vi "crio_RT_Antagonist_Precision.vi"() -> ()   [LabVIEW 2019]
uses:
  <vilib>/Platform/TimedLoop/XDataNode/timing_clust.ctl
  <vilib>/Platform/TimedLoop/XDataNode/nitl_modes.ctl
  <vilib>/Platform/TimedLoop/XDataNode/wakeup.ctl
  <vilib>/FPGAPlugInAG/cRIO-9074/niLvFpga_Open_cRIO-9074.vi
  <vilib>/rvi/interface/common/dynamic/niFpgaDynamicAddResources.vi
  <vilib>/Utility/file.llb/Write Delimited Spreadsheet (string).vi
  <vilib>/Utility/error.llb/Error Cluster From Error Code.vi
  <vilib>/rvi/errors/niLvFpgaAdjustHostInterfaceError.vi
  <vilib>/FPGAPlugInAG/Dynamic/niLvFpga_Close_Dynamic.vi
  <vilib>/rvi/interface/nirviOpenFPGA/nirviOpenFPGA.xnode
  FPGA Bitfiles/gpass2_FPGATarget2_crioFPGAAntagoni_cDOKBUczdNQ.lvbitx
  crio_FPGA_Antagonist_Radial.vi
  <vilib>/rvi/interface/nirviReadWriteControl/nirviReadWriteControl.xnode
  <vilib>/platform/TimedLoop/XDataNode/XDataNode.xnode
  <vilib>/rvi/interface/nirviCloseFPGA/nirviCloseFPGA.xnode
  NiFpgaLv.dll
  <vilib>/rvi/interface/Simulation/niFpgaSimulationCallBeginRW.vi
  <vilib>/Platform/TimedLoop/XDataNode/XDNodeRunTimeDep.lvlib
  <vilib>/Utility/file.llb/Write Delimited Spreadsheet (I64).vi
panel:
  out "appended array":i32[](array[numeric])
  in  "precision test .csv name":string="precision_test.csv"
  in  "Channel Names":string[](array[string])=["Channel 1", "Channel 2", "Channel 3", "Channel 4", "Channel 5"]
  out "log file path":path
  out "error out":errorcluster
  in  "Header Info":string[][](array[string])=[["Test Name", "Operator", "UUT"], ["Voltage", "National Instruments", "AA123"]]
  in  "mSec to take Sample":u32
  in  "LAC Full Extract Position":i32(slide) scale=0.0..4500.0
  in  "VCA Full Extract Position":i32(slide) scale=0.0..2700.0
  in  "Rail Full Extract Position":i16(slide) scale=0.0..20000.0
  out "VCA Setpoint":i32
  out "Rail Setpoint":i16
  out "LAC Setpoint":i32
  in  "Start Test":bool
  out "Rail Position":i16(graph)
  out "rail Platform Position":i16
  in  "Half Peirod (pulse 40MHz)":u32=10000
  in  "Rail Stepper Direction":bool
  in  "Rail Stepper Enable":bool
  in  "Rail Manual Operation":bool
  in  "Autolock":bool
  out "LAC Measured Position":i32(graph)
  out "LAC Measured Position":i32
  in  "LAC manual control":T1={"manual? (F)"=FALSE, "manual input (0)"=-0.83838385} {"manual input (0)" scale=-1.0..1.0}
  in  "LAC Position Reset":bool
  in  "LAC Gains":T2={"proportional gain"=0.95454544, "integral gain"=0.4949495} {"proportional gain" scale=0.0..1.0; "integral gain" scale=0.0..1.0}
  in  "LAC Velocity Interval (uSec)":u32=1000
  out "LAC Actual Gain":T2={"proportional gain"=0.009545455, "integral gain"=1.2626262e-09}
  in  "LAC Gain Scaler":T2={"proportional gain"=100.0, "integral gain"=100000000.0}
  in  "stop":bool
  out "VCA Measured Velocity (Counts/Interval)":i32
  out "VCA Controller PWM Output":sgl=-0.35149753
  out "VCA Measured Position":i32=4
  in  "VCA Loop Period(us)":i64=2000
  out "VCA Measured Position":i32(graph)=4
  in  "VCA  manual control":T1 {"manual input (0)" scale=-1.0..1.0}
  in  "VCA Position Reset":bool
  in  "VCA Gains":T2={"proportional gain"=0.97979796, "integral gain"=0.7979798} {"proportional gain" scale=0.0..1.0; "integral gain" scale=0.0..1.0}
  in  "VCA Velocity Interval (uSec)":u32=1000
  out "VCA Actual Gain":T2={"proportional gain"=0.0009797979, "integral gain"=7.979798e-09}
  in  "VCA Gain Scaler":T2={"proportional gain"=1000.0, "integral gain"=100000000.0}
  in  "PWM Frequency (default 20kHz)":i32=20000
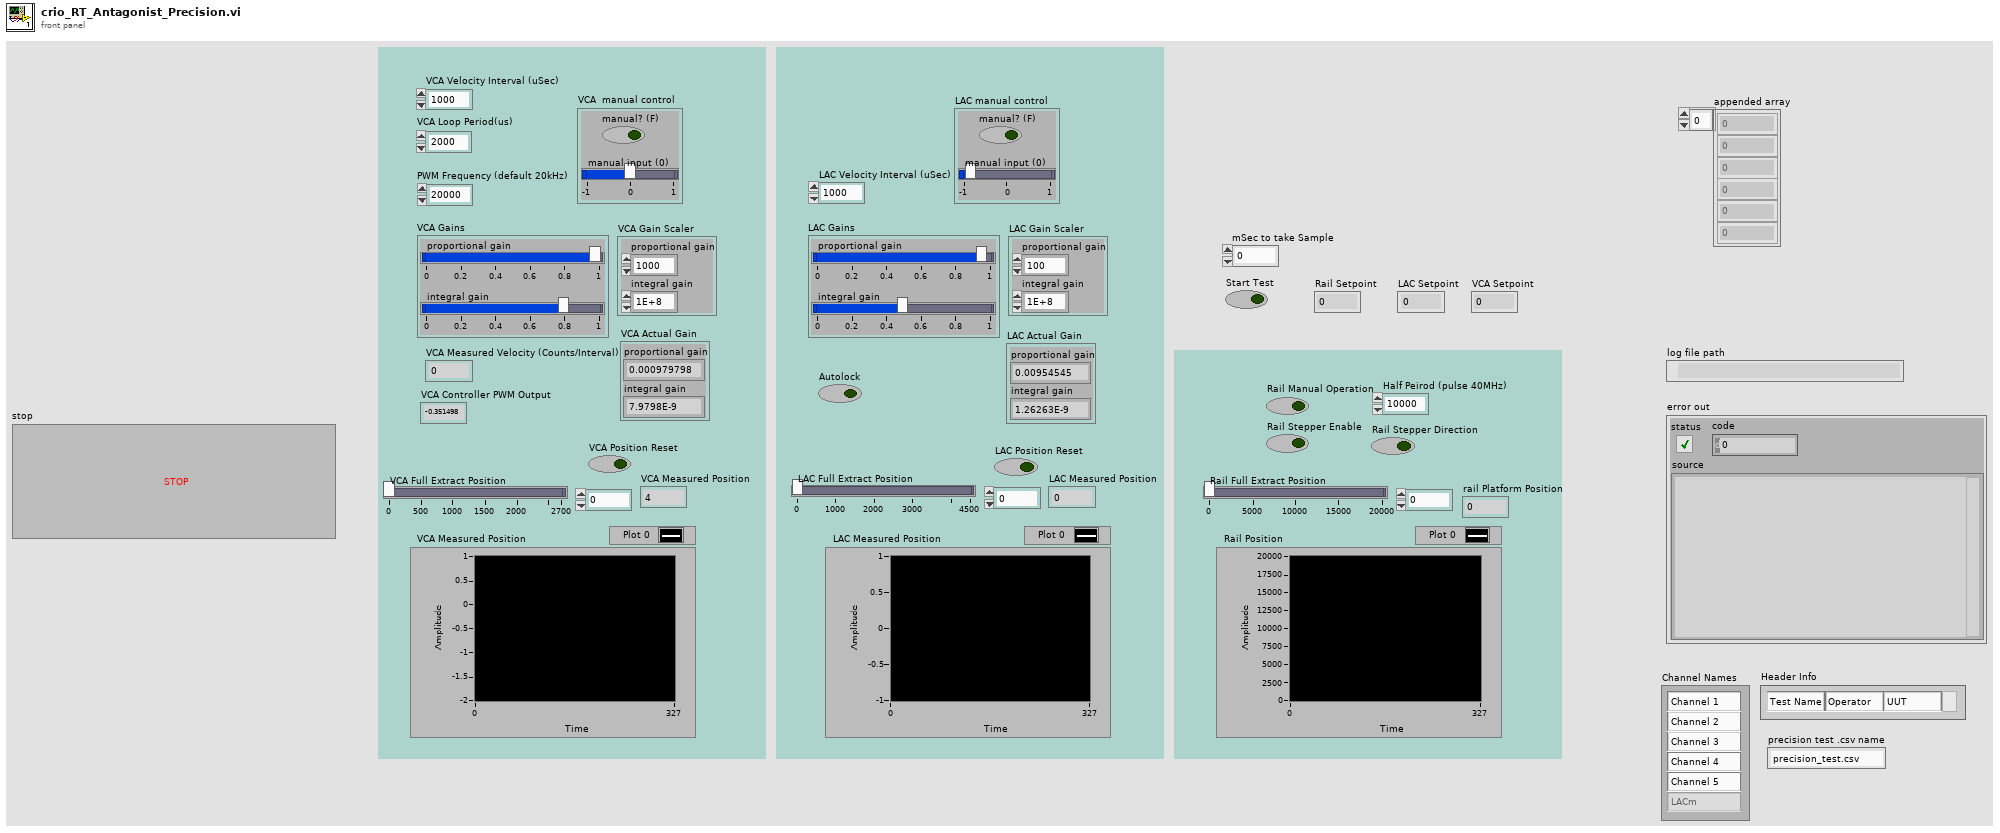
[diagram p1: front panel]
types:
  T1 = cluster{"manual? (F)":bool, "manual input (0)":sgl}
  T2 = cluster{"proportional gain":sgl, "integral gain":sgl}
  T3 = typedef "XDNodeRunTimeDep.lvlib/timing_clust.ctl" = cluster{"Expected End [f-1]":u64, "Actual End [f-1]":u64, "Finished Late? [f-1]":bool, "Expected End [i-1]":u64, "Actual End [i-1]":u64, "Finished Late? [i-1]":bool, "Expected Start [i]":u64, "Actual Start [i]":u64, "Expected Start [f]":u64, "Actual Start [f]":u64, "Source Name":string, "Structure Name":string, "Period":i64, "Deadline":i64, "Offset":i64, "Start":i64, "Priority":i32, "Timeout":i32, "Mode":T4, "Wakeup Reason":T5, "Error":errorcluster, "Source Type":string, "Secondary Source Type":string, "Global End Time":u64, "Global Start Time":u64, "Frame Duration":u64, "Iteration Duration":u64, "Assigned CPU":i32, "I/O Scan Engine Mode":u32}
  T4 = typedef "XDNodeRunTimeDep.lvlib/nitl_modes.ctl" = enum32{"No Change", "Process missed periods, maintain original phase", "Discard missed periods, maintain original phase", "Process missed periods, ignore original phase", "Discard missed periods, ignore original phase"}
  T5 = typedef "XDNodeRunTimeDep.lvlib/wakeup.ctl" = enum32{"Normal", "Aborted", "Asynchronous wakeup", "Timing source error", "Timed loop error", "Timeout"}
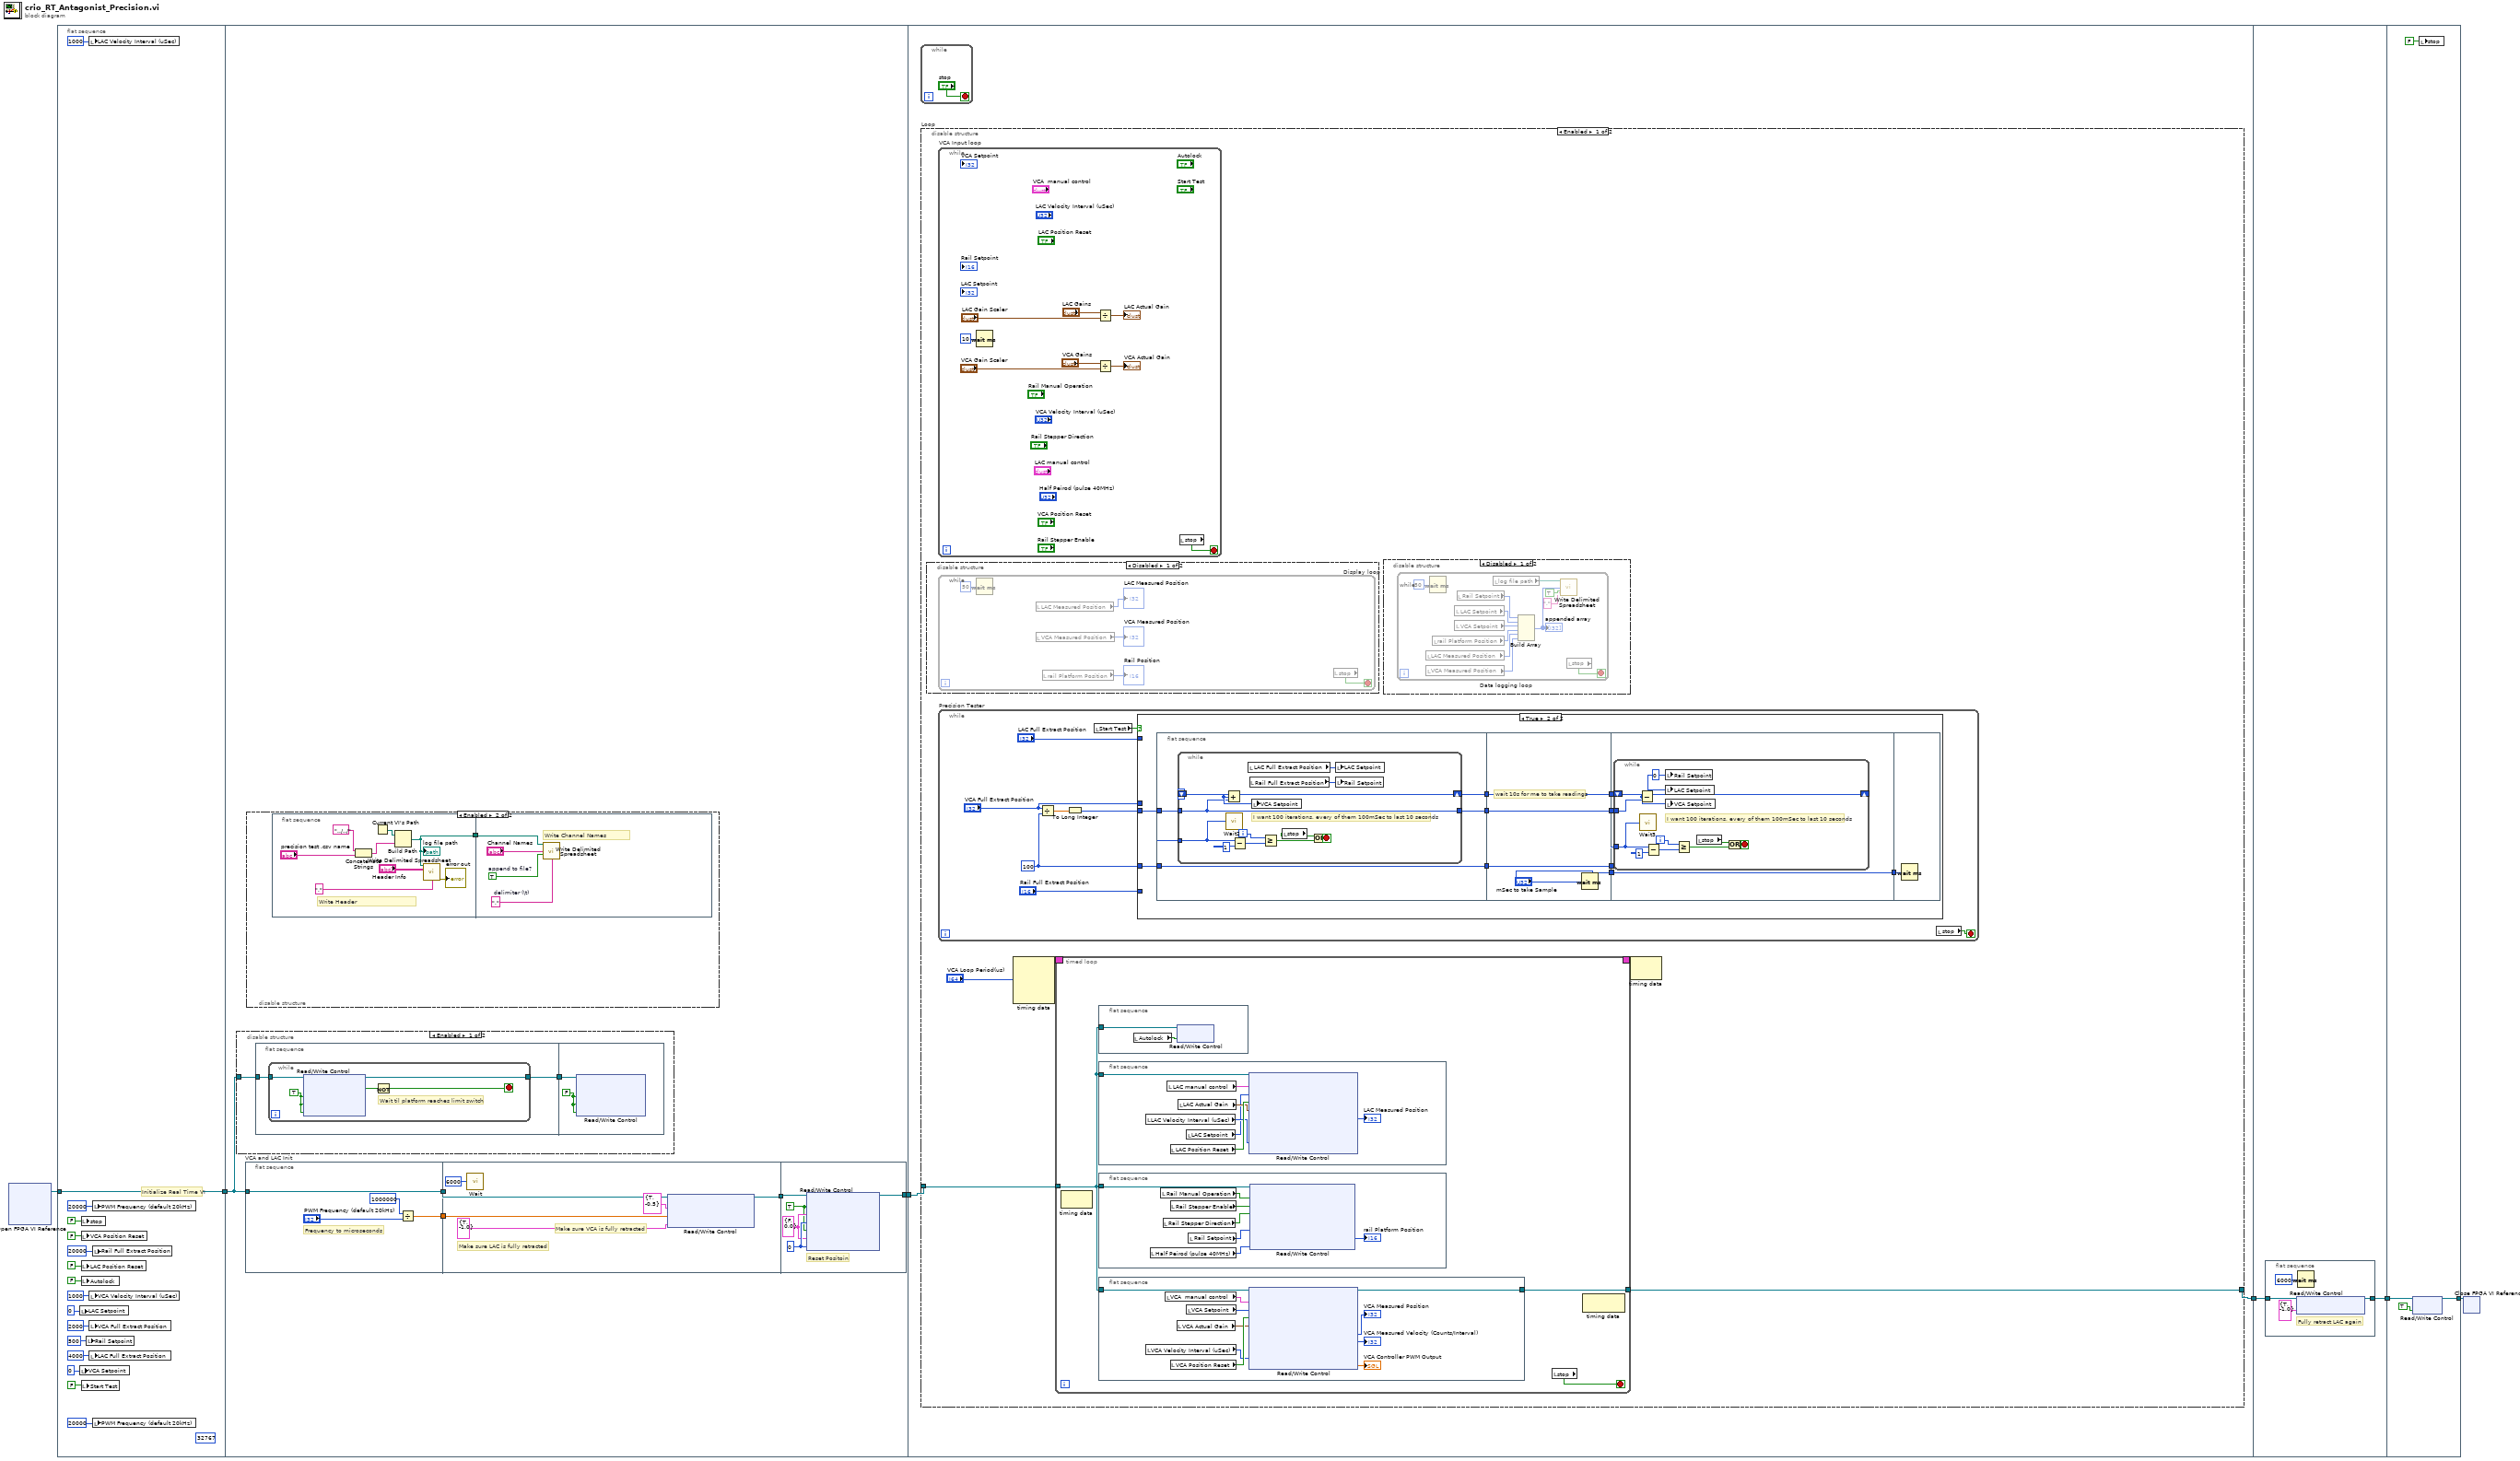
[diagram p0: block diagram]
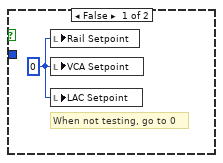
[diagram p6: hidden frame]
diagram:
  n1 = xnode "Open FPGA VI Reference"() -> ("FPGA VI Reference Out"=w6:refnum<k20>)  [unwired: 2 in, 1 out]
  n2 = flat-sequence {
    tunnel: w6 -> [w21]
    tunnel: [w21] -> w5
    tunnel: [w27] -> w4
    tunnel: w5 -> [w23]
    tunnel: w4 -> [w68]
    tunnel: [w67] -> w2
    tunnel: w2 -> [w192]
    tunnel: [w191] -> w1
    tunnel: w1 -> [w200]
    tunnel: [w199] -> w3
    frame #0 {
      (unwired) i16 32767 ("Initialize Rail Position")
      # "Initialize Real Time VI"
      n3 = local write "LAC Setpoint"(0 ("VCA setpoint")) -> ()
      n4 = local write "VCA Setpoint"(0 ("VCA setpoint")) -> ()
      n5 = local write "stop"(FALSE ("stop")) -> ()
      n6 = local write "VCA Position Reset"(FALSE ("VCA Position Reset")) -> ()
      n7 = local write "LAC Position Reset"(FALSE ("VCA Position Reset")) -> ()
      n8 = local write "Autolock"(FALSE ("Autolock")) -> ()
      n9 = local write "Start Test"(FALSE ("Test Precision")) -> ()
      n10 = local write "Rail Setpoint"(i16 500 ("Rail Desired Position")) -> ()
      n11 = local write "LAC Velocity Interval (uSec)"(u32 1000 ("Velocity Interval (uSec)")) -> ()
      n12 = local write "VCA Velocity Interval (uSec)"(u32 1000 ("Velocity Interval (uSec)")) -> ()
      n13 = local write "VCA Full Extract Position"(2000 ("VCA setpoint")) -> ()
      n14 = local write "LAC Full Extract Position"(4000 ("VCA setpoint")) -> ()
      n15 = local write "PWM Frequency (default 20kHz)"(20000 ("PWM Frequency (default 20kHz)")) -> ()
      n16 = local write "Rail Full Extract Position"(20000 ("VCA setpoint")) -> ()
      n17 = local write "PWM Frequency (default 20kHz)"(20000 ("PWM Frequency")) -> ()
    }
    frame #1 {
      n18 = disable-structure shown="Enabled" {
        disable-tunnel: w23 -> [w41 _]
        frame Enabled {
          n19 = flat-sequence {
            tunnel: w41 -> [w43]
            tunnel: [w44] -> w42
            tunnel: w42 -> [w51]
            frame #0 {
              n20 = while {
                tunnel: [w48] -> w44
                tunnel: w43 -> [w47]
                stop <- w45 stop-if-true
                w49 = TRUE ("Stepper Direction")
                # "Wait til platform reaches limit switch"
                n21 = xnode "Read/Write Control"("FPGA VI Reference In"=w47, "Manual Operation"=w49, "Stepper Enable"=w49, "Stepper Direction"=w49) -> ("FPGA VI Reference Out"=w48:refnum<k20>, "Limit Switch"=w46:bool)  [unwired: 1 in, 1 out]
                n22 = Not(x=w46) -> (.not. x?=w45:bool)
              }
            }
            frame #1 {
              w50 = FALSE ("Stepper Direction")
              n23 = xnode "Read/Write Control"("FPGA VI Reference In"=w51, "Manual Operation"=w50, "Stepper Enable"=w50, "Stepper Direction"=w50) -> ()  [unwired: 1 in, 3 out]
            }
          }
        }
        frame Disabled {
        }
      }
      n24 = flat-sequence "VCA and LAC Init" {
        tunnel: [w54] -> w26
        tunnel: w23 -> [w52]
        tunnel: [w52] -> w25
        tunnel: w26 -> [w60]
        tunnel: w25 -> [w56]
        tunnel: [w61] -> w24
        tunnel: w24 -> [w65]
        tunnel: [w66] -> w27
        frame #0 {
          # "Frequency to microseconds"
          n25 = Divide(x=1000000, y="PWM Frequency (default 20kHz)") -> (x/y=w54:dbl)
        }
        frame #1 {
          # "Make sure LAC is fully retracted"
          # "Make sure VCA is fully retracted"
          n26 = call "Wait"("Count(mSec)"=u32 6000) -> ()  [unwired: 1 out]
          n27 = xnode "Read/Write Control"("FPGA VI Reference In"=w56, "VCA Manual Control"=T1 {"manual? (F)"=TRUE, "manual input (0)"=-0.5} ("manual control"), "DC PWM Period (microsec)"=w60, "LAC Manual Control"=T1 {"manual? (F)"=TRUE, "manual input (0)"=-1.0} ("manual control")) -> ("FPGA VI Reference Out"=w61:refnum<k20>)  [unwired: 1 in, 1 out]
        }
        frame #2 {
          w64 = 0 ("setpoint")
          w63 = T1 {"manual? (F)"=FALSE, "manual input (0)"=0.0} ("manual control")
          w62 = TRUE ("Position Reset")
          # "Reset Positoin"
          n28 = xnode "Read/Write Control"("FPGA VI Reference In"=w65, "VCA Position Reset"=w62, "VCA Manual Control"=w63, "VCA Position Setpoint"=w64, "Position Reset"=w62, "LAC Manual Control"=w63, "LAC Setpoint"=w64) -> ("FPGA VI Reference Out"=w66:refnum<k20>)  [unwired: 1 in, 1 out]
        }
      }
      n29 = disable-structure shown="Enabled" {
        frame Disabled {
        }
        frame Enabled {
          n30 = flat-sequence {
            tunnel: [w32] -> w28
            tunnel: w28 -> [w37]
            frame #0 {
              # "Write Header"
              n31 = Concatenate Strings("../../" ("name or relative path"), "precision test .csv name") -> (w29:string)
              n32 = Current VI's Path() -> (path=w33:path)
              n33 = Build Path(base path=w33, name or relative path=w29) -> (appended path=w32:path)
              "log file path" <- w32
              n34 = call-poly <vilib>:"Write Delimited Spreadsheet.vi"("file path (dialog if empty)"=w32, "2D data"="Header Info", "delimiter (\\t)"="," ("delimiter (\\t)")) -> ("error out"=→"error out":errorcluster)  [unwired: 11 in, 1 out]
            }
            frame #1 {
              w39 = TRUE  # append to file?
              w38 = ","  # delimiter (\t)
              # "Write Channel Names"
              n35 = call-poly <vilib>:"Write Delimited Spreadsheet.vi"("file path (dialog if empty)"=w37, "1D data"="Channel Names", "append to file? (new file:F)"=w39, "delimiter (\\t)"=w38) -> ()  [unwired: 10 in, 2 out]
            }
          }
        }
      }
    }
    frame #2 {
      n36 = while {
        stop <- "stop" stop-if-true
      }
      n37 = disable-structure "Loop" shown="Enabled" {
        disable-tunnel: w68 -> [w70 _]
        disable-tunnel: [w69 _] -> w67
        frame Enabled {
          n38 = disable-structure shown="Disabled" {
            frame Disabled {
              n39 = while "Display loop" {
                stop <- w89 stop-if-true
                n40 = Wait (ms)(milliseconds to wait=u32 50) -> ()  [unwired: 1 out]
                n41 = local read "LAC Measured Position"() -> (→"LAC Measured Position":i32)
                n42 = local read "VCA Measured Position"() -> (→"VCA Measured Position":i32)
                n43 = local read "rail Platform Position"() -> (→"Rail Position":i16)
                n44 = local read "stop"() -> (w89:bool)
              }
            }
            frame Enabled {
            }
          }
          n45 = while "VCA Input loop" {
            stop <- w153 stop-if-true
            n46 = Wait (ms)(milliseconds to wait=u32 10) -> ()  [unwired: 1 out]
            n47 = Divide(x="LAC Gains", y="LAC Gain Scaler") -> (x/y=→"LAC Actual Gain":T2)
            n48 = Divide(x="VCA Gains", y="VCA Gain Scaler") -> (x/y=→"VCA Actual Gain":T2)
            n49 = local read "stop"() -> (w153:bool)
          }
          n50 = while "Precision Tester" {
            stop <- w98 stop-if-true
            w95 = i16 100 ("y")
            n51 = Divide(x="VCA Full Extract Position", y=w95) -> (x/y=w94:dbl)
            n52 = To Long Integer(number=w94) -> (32bit integer=w93:i32)
            n53 = local read "Start Test"() -> (w97:bool)
            n54 = case shown="True" w97 {
              tunnel: "Rail Full Extract Position" -> [_ _]
              tunnel: w95 -> [_ w109]
              tunnel: w93 -> [_ w104]
              tunnel: "VCA Full Extract Position" -> [_ _]
              tunnel: "LAC Full Extract Position" -> [_ _]
              frame False {
                w99 = i16 0 ("Rail Setpoint")
                # "When not testing, go to 0"
                n55 = local write "Rail Setpoint"(w99) -> ()
                n56 = local write "VCA Setpoint"(w99) -> ()
                n57 = local write "LAC Setpoint"(w99) -> ()
              }
              frame True {
                n58 = flat-sequence {
                  tunnel: w109 -> [w114]
                  tunnel: [w114] -> w106
                  tunnel: w104 -> [w112]
                  tunnel: [w111] -> w102
                  tunnel: [w110] -> w100
                  tunnel: ["mSec to take Sample"] -> w107
                  tunnel: w106 -> [w129]
                  tunnel: [w129] -> w105
                  tunnel: [w128] -> w103
                  tunnel: w102 -> [w128]
                  tunnel: [w127] -> w101
                  tunnel: w100 -> [w127]
                  tunnel: [w134] -> w108
                  tunnel: w107 -> [w134]
                  tunnel: w105 -> [w133]
                  tunnel: w103 -> [w132]
                  tunnel: w101 -> [w131]
                  tunnel: w108 -> [w146]
                  frame #0 {
                    n59 = while {
                      tunnel: w114 -> [w122]
                      shift-right: [w118] -> w111
                      shift-left: 0 ("milliseconds to wait") -> [w117]
                      tunnel: w112 -> [w116]
                      tunnel: [w116] -> w110
                      i -> [w123]
                      stop <- w125 stop-if-true
                      # "I want 100 iterations, every of them 100mSec to last 10 seconds"
                      n60 = Add(x=w117, y=w116) -> (x+y=w118:i32)
                      n61 = call "Wait2"("Count(mSec)"=w122) -> ()  [unwired: 1 out]
                      n62 = Subtract(x=w122, y=i16 1) -> (x-y=w120:i16)
                      n63 = local read "LAC Full Extract Position"() -> (w115:i32)
                      n64 = local read "Rail Full Extract Position"() -> (w119:i16)
                      n65 = local write "VCA Setpoint"(w118) -> ()
                      n66 = Greater Or Equal?(x=w123, y=w120) -> (x >= y?=w124:bool)
                      n67 = local read "stop"() -> (w126:bool)
                      n68 = Or(x=w126, y=w124) -> (x .or. y?=w125:bool)
                      n69 = local write "LAC Setpoint"(w115) -> ()
                      n70 = local write "Rail Setpoint"(w119) -> ()
                    }
                  }
                  frame #1 {
                    # "wait 10s for me to take readings"
                    n71 = Wait (ms)(milliseconds to wait="mSec to take Sample") -> ()  [unwired: 1 out]
                  }
                  frame #2 {
                    n72 = while {
                      tunnel: w133 -> [w141]
                      shift-right: [w138] -> _
                      shift-left: w132 -> [w137]
                      tunnel: w131 -> [w136]
                      i -> [w143]
                      stop <- w144 stop-if-true
                      w135 = i16 0 ("Rail Setpoint")
                      # "I want 100 iterations, every of them 100mSec to last 10 seconds"
                      n73 = Subtract(x=w137, y=w136) -> (x-y=w138:i32)
                      n74 = call "Wait3"("Count(mSec)"=w141) -> ()  [unwired: 1 out]
                      n75 = Subtract(x=w141, y=i16 1) -> (x-y=w139:i16)
                      n76 = local write "Rail Setpoint"(w135) -> ()
                      n77 = local write "LAC Setpoint"(w135) -> ()
                      n78 = local write "VCA Setpoint"(w138) -> ()
                      n79 = Greater Or Equal?(x=w143, y=w139) -> (x >= y?=w142:bool)
                      n80 = local read "stop"() -> (w145:bool)
                      n81 = Or(x=w145, y=w142) -> (x .or. y?=w144:bool)
                    }
                  }
                  frame #3 {
                    n82 = Wait (ms)(milliseconds to wait=w146) -> ()  [unwired: 1 out]
                  }
                }
              }
            }
            n83 = local read "stop"() -> (w98:bool)
          }
          n84 = node-c288("VCA Loop Period(us)") -> (w73:T3)  [unwired: 3 in]
          n85 = timed-loop {
            timing: w73 -> [_]
            timing-out: [_] -> w72
            tunnel: w70 -> [w155]
            tunnel: [w157] -> w69
            stop <- w156 stop-if-true
            n86 = node-c288() -> ()  [unwired: 1 in, 1 out]
            n87 = flat-sequence {
              tunnel: w155 -> [w166]
              frame #0 {
                n88 = local read "Autolock"() -> (w165:bool)
                n89 = xnode "Read/Write Control"("FPGA VI Reference In"=w166, "LAC Lock"=w165) -> ()  [unwired: 1 in, 2 out]
              }
            }
            n90 = flat-sequence {
              tunnel: w155 -> [w173]
              frame #0 {
                n91 = local read "LAC Velocity Interval (uSec)"() -> (w169:u32)
                n92 = local read "LAC manual control"() -> (w172:T1)
                n93 = local read "LAC Position Reset"() -> (w171:bool)
                n94 = local read "LAC Actual Gain"() -> (w170:T2)
                n95 = local read "LAC Setpoint"() -> (w167:i32)
                n96 = xnode "Read/Write Control"("FPGA VI Reference In"=w173, "LAC Manual Control"=w172, "LAC Setpoint"=w167, "Position Reset"=w171, "LAC Gains"=w170, "LAC Velocity Interval (uSec)"=w169) -> ("LAC Position (Counts)"=→"LAC Measured Position":i32)  [unwired: 1 in, 5 out]
              }
            }
            n97 = flat-sequence {
              tunnel: w155 -> [w159]
              frame #0 {
                n98 = local read "Half Peirod (pulse 40MHz)"() -> (w164:u32)
                n99 = local read "Rail Manual Operation"() -> (w161:bool)
                n100 = local read "Rail Stepper Direction"() -> (w162:bool)
                n101 = local read "Rail Stepper Enable"() -> (w163:bool)
                n102 = local read "Rail Setpoint"() -> (w158:i16)
                n103 = xnode "Read/Write Control"("FPGA VI Reference In"=w159, "Manual Operation"=w161, "Stepper Enable"=w163, "Stepper Direction"=w162, "Position Control: Desired Positoin"=w158, "Half Peirod (pulse 40MHz)"=w164) -> ("rail Platform Position"=→"rail Platform Position":i16)  [unwired: 2 in, 2 out]
              }
            }
            n104 = flat-sequence {
              tunnel: [w176] -> w157
              tunnel: w155 -> [w175]
              frame #0 {
                n105 = local read "VCA Velocity Interval (uSec)"() -> (w174:u32)
                n106 = local read "VCA  manual control"() -> (w177:T1)
                n107 = local read "VCA Position Reset"() -> (w180:bool)
                n108 = local read "VCA Actual Gain"() -> (w179:T2)
                n109 = local read "VCA Setpoint"() -> (w178:i32)
                n110 = xnode "Read/Write Control"("FPGA VI Reference In"=w175, "VCA Manual Control"=w177, "VCA Position Setpoint"=w178, "VCA Position Reset"=w180, "VCA Gains"=w179, "Velocity Interval (uSec)"=w174) -> ("FPGA VI Reference Out"=w176:refnum<k20>, "Position (Counts) VCA"=→"VCA Measured Position":i32, "Velocity (Counts/Interval) VCA"=→"VCA Measured Velocity (Counts/Interval)":i32, "VCA ControllerPWM Output"=→"VCA Controller PWM Output":sgl)  [unwired: 1 in, 2 out]
              }
            }
            n111 = local read "stop"() -> (w156:bool)
            n112 = node-c288() -> ()  [unwired: 1 in, 1 out]
          }
          n113 = disable-structure shown="Disabled" {
            frame Disabled {
              n114 = while "Data logging loop" {
                stop <- w84 stop-if-true
                n115 = local read "LAC Measured Position"() -> (w79:i32)
                n116 = local read "VCA Measured Position"() -> (w78:i32)
                n117 = Wait (ms)(milliseconds to wait=u32 50) -> ()  [unwired: 1 out]
                n118 = local read "rail Platform Position"() -> (w80:i16)
                n119 = local read "LAC Setpoint"() -> (w82:i32)
                n120 = local read "VCA Setpoint"() -> (w81:i32)
                n121 = local read "Rail Setpoint"() -> (w83:i16)
                n122 = local read "log file path"() -> (w74:path)
                n123 = Build Array(w83, w82, w81, w80, w79, w78) -> (w75:i32[])
                "appended array" <- w75
                n124 = call-poly <vilib>:"Write Delimited Spreadsheet.vi"("file path (dialog if empty)"=w74, "1D data"=w75, "append to file? (new file:F)"=TRUE, "delimiter (\\t)"="," ("delimiter (\\t)")) -> ()  [unwired: 10 in, 2 out]
                n125 = local read "stop"() -> (w84:bool)
              }
            }
            frame Enabled {
            }
          }
          n126 = node-c288(w72) -> ()  [unwired: 1 out]
        }
        frame Disabled {
        }
      }
    }
    frame #3 {
      n127 = flat-sequence {
        tunnel: w192 -> [w195]
        tunnel: [w194] -> w191
        frame #0 {
          # "Fully retract LAC again"
          n128 = xnode "Read/Write Control"("FPGA VI Reference In"=w195, "LAC Manual Control"=T1 {"manual? (F)"=TRUE, "manual input (0)"=-1.0}) -> ("FPGA VI Reference Out"=w194:refnum<k20>)  [unwired: 1 in, 1 out]
          n129 = Wait (ms)(milliseconds to wait=u32 6000) -> ()  [unwired: 1 out]
        }
      }
    }
    frame #4 {
      n130 = xnode "Read/Write Control"("FPGA VI Reference In"=w200, "stop"=TRUE) -> ("FPGA VI Reference Out"=w199:refnum<k20>)  [unwired: 1 in, 1 out]
      n131 = local write "stop"(FALSE ("stop")) -> ()
    }
  }
  n132 = xnode "Close FPGA VI Reference"("FPGA VI Reference In"=w3) -> ()  [unwired: 1 in, 1 out]
